vi "Publish Results.vi"(8 "error in (no error)":errorcluster, 10 "Results":T1[](array[typedef]), 11 "LUnit Test Case V2 In":refnum<class "LUnit Test Case V2.lvclass">) -> (0 "error out":errorcluster, 3 "LUnit Test Case V2 Out":refnum<class "LUnit Test Case V2.lvclass">)   [LabVIEW 2020, in "LUnit Test Case V2.lvclass"]
uses:
  LUnit Test Case V2.lvclass
  Result/Result.ctl
  Result/Status.ctl
  Result/Type.ctl
  LUnit Test Case V2.lvclass/LUnit Test Case V2.ctl
  Result Observer/Result Observer.lvclass
  Result/Result.lvlib
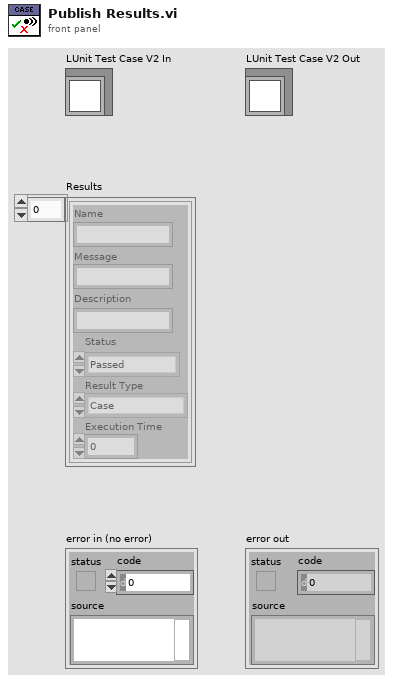
[diagram p1: front panel]
types:
  T1 = typedef "Result.lvlib/Result.ctl" = cluster{"Name":string, "Message":string, "Description":string, "Status":T2, "Result Type":T3, "Execution Time":dbl}
  T2 = typedef "Result.lvlib/Status.ctl" = enum16{"", "Passed", "Failed", "Error", "Skipped", "Setup Error", "Broken", "Teardown Error"}
  T3 = typedef "Result.lvlib/Type.ctl" = enum16{"Method", "Case", "Suite", "Pass", "Fail", "Skip", "Pass if", "Fail if", "Pass if Error", "Fail if Error", "Pass if Equal", "Fail if Equal"}
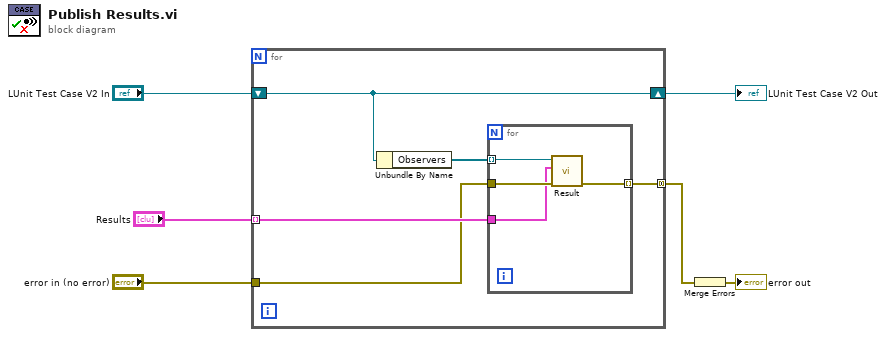
[diagram p0: block diagram]
diagram:
  n1 = for {
    tunnel: "Results" -> [w10] mode=indexing
    tunnel: "error in (no error)" -> [w9]
    tunnel: [w8] -> w3 mode=concatenating
    shift-right: [w7] -> w2
    shift-left: "LUnit Test Case V2 In" -> [w7]
    n2 = Unbundle By Name(w7) -> ("Observers"=w11:refnum<class "Result Observer.lvclass">[])
    n3 = for {
      tunnel: w11 -> [w15] mode=indexing
      tunnel: w9 -> [w14]
      tunnel: w10 -> [w13]
      tunnel: [w12] -> w8 mode=indexing
      n4 = call-dynamic "Result.vi"("error in (no error)"=w14, "Result"=w13, "Result Observer in"=w15) -> ("error out"=w12:errorcluster)  [unwired: 8 in]
    }
  }
  "LUnit Test Case V2 Out" <- w2
  n5 = Merge Errors(w3) -> (→"error out":errorcluster)
